vi "CLAD 5-3.vi"() -> ()   [LabVIEW 2014]
uses:
  Type Def Numeric.ctl
  Def Numeric.ctl
panel:
  in  "Type Def Numeric":T1
  in  "Strict Type Def Numeric":T2
  # "I was able to change the different controls back and forth and see how editing them works"
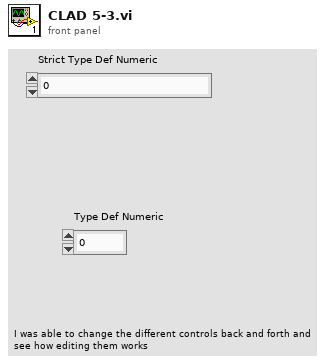
[diagram p1: front panel]
types:
  T1 = typedef "Def Numeric.ctl" = dbl
  T2 = typedef "Type Def Numeric.ctl" = dbl
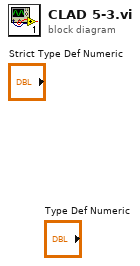
[diagram p0: block diagram]
diagram:
